vi "Wait for Trigger.vi"(8 "error in (no error)":errorcluster, 11 "rfsg queue":refnum<queue>) -> (0 "error out":errorcluster, 3 "abort?":bool)   [LabVIEW 2021]
uses:
  RFSG Configuration.ctl
  Messaging/RFSG Message.ctl
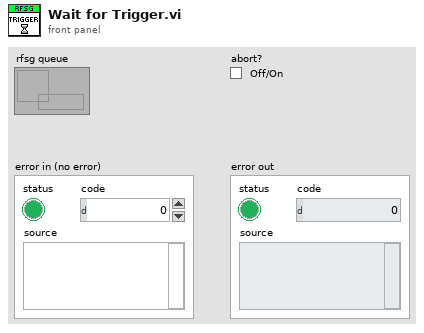
[diagram p1: front panel]
types:
  T1 = typedef "RFSG Message.ctl" = enum16{"Trigger Ready", "Run RF", "Stop RF", "Exit"}
  T2 = typedef "RFSG Configuration.ctl" = cluster{"rfsg ref":refnum<k15>, "freq off":i32, "wfm type":u16, "cent freq":dbl, "iq rate":dbl, "power":dbl, "msg":T1}
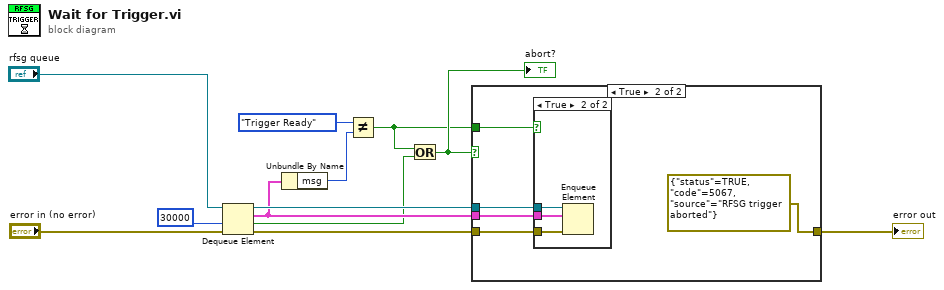
[diagram p0: block diagram]
diagram:
  n1 = Dequeue Element(queue="rfsg queue", timeout in ms (-1)=30000, error in (no error)="error in (no error)") -> (queue out=w5:refnum<queue>, element=w4:T2, timed out?=w3:bool, error out=w7:errorcluster)
  n2 = Unbundle By Name(w4) -> ("msg"=w9:T1)
  n3 = Not Equal?(x=RFSG_Message."Trigger Ready", y=w9) -> (x != y?=w1:bool)
  n4 = Or(x=w1, y=w3) -> (x .or. y?=w2:bool)
  "abort?" <- w2
  n5 = case shown="True" w2 {
    tunnel: w7 -> [w13 w18]
    tunnel: [w13 errorcluster {"status"=TRUE, "code"=5067, "source"="RFSG trigger aborted"} ("error out")] -> w6
    tunnel: w5 -> [_ w17]
    tunnel: w4 -> [_ w16]
    tunnel: w1 -> [_ w14]
    frame False {
    }
    frame True {
      n6 = case shown="True" w14 {
        tunnel: w18 -> [_ w21]
        tunnel: w17 -> [_ w20]
        tunnel: w16 -> [_ w19]
        frame False {
        }
        frame True {
          n7 = Enqueue Element(queue=w20, element=w19, error in (no error)=w21) -> ()  [unwired: 1 in, 3 out]
        }
      }
    }
  }
  "error out" <- w6
